vi "ReadoutQx.vi"(2 "error in":errorcluster, 3 "address string":string="19") -> (0 "error out":errorcluster, 1 "String":string)   [LabVIEW 2010]
panel:
  in  "mode (0) 2":i16
  in  "mode (0)":i16
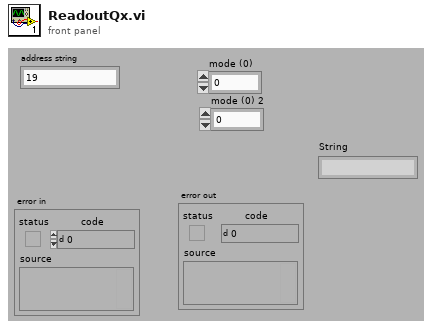
[diagram p1: front panel]
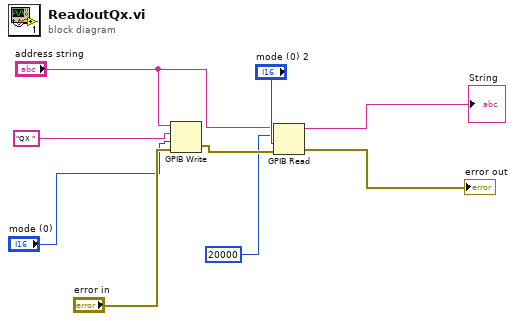
[diagram p0: block diagram]
diagram:
  n1 = GPIB Write(0:"address string", 1:"QX ", 2:"mode (0)", 3:"error in") -> (6:w7:errorcluster)  [unwired: 1 in, 1 out]
  n2 = GPIB Read(0:"address string", 1:20000, 2:"mode (0) 2", 3:w7) -> (5:→"String":string, 7:→"error out":errorcluster)  [unwired: 1 in, 1 out]
